vi "Unconstrained Logarithm Fit.vi"(0 "Y":dbl[](array[numeric]), 1 "base":dbl(ring)=2.71828 items=["e"=2.71828, "2"=2.0, "10"=10.0], 5 "X":dbl[](array[numeric]), 7 "Weight":dbl[](array[numeric]), 9 "tolerance":dbl=0.0001, 11 "method":T1 items=["Least Square", "Least Absolute Residual", "Bisquare"]) -> (4 "Best Logarithm Fit":dbl[](array[numeric]), 6 "amplitude":dbl, 8 "scale":dbl, 14 "residue":dbl, 15 "error":i32)   [LabVIEW 2017, in "NI_AALPro.lvlib"]
doc: "Returns the logarithmic fit of a data set (<B>X</B>, <B>Y</B>) using the Least Square, Least Absolute Residual, or Bisquare method."
uses:
  <vilib>/Analysis/NI_AALPro.lvlib
  <vilib>/Analysis/6fits.llb/Curve Fitting Criteria.ctl
panel:
  # "Logarithm Fit"
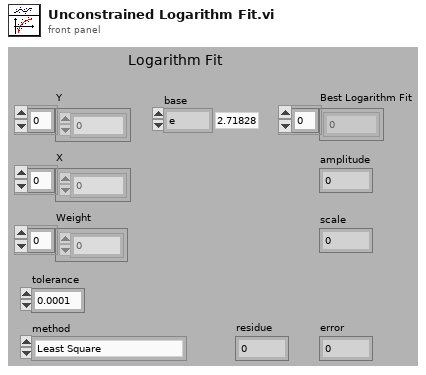
[diagram p1: front panel]
types:
  T1 = typedef "NI_AALPro.lvlib/Curve Fitting Criteria.ctl" = u16
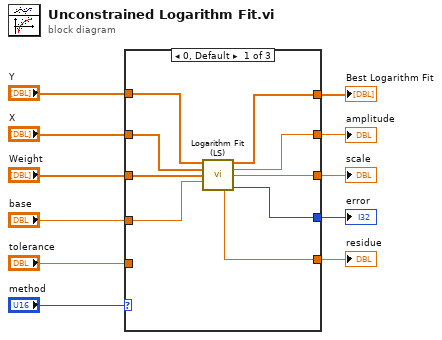
[diagram p0: block diagram]
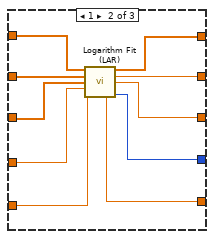
[diagram p2: hidden frame]
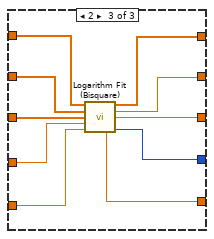
[diagram p3: hidden frame]
diagram:
  n1 = case shown="0, Default" "method" {
    tunnel: "Y" -> [w20 w30 w40]
    tunnel: "X" -> [w19 w29 w39]
    tunnel: "Weight" -> [w18 w28 w38]
    tunnel: "base" -> [w17 w27 w37]
    tunnel: [w16 w25 w35] -> w6
    tunnel: [w15 w24 w34] -> w5
    tunnel: [w14 w23 w33] -> w4
    tunnel: [w13 w22 w32] -> w3
    tunnel: [w12 w21 w31] -> w2
    tunnel: "tolerance" -> [_ w26 w36]
    frame 0, Default {
      n2 = call <vilib>:"Logarithm Fit (LS).vi"("Y"=w20, "X"=w19, "Weight"=w18, "base of logarithm"=w17) -> ("Best Logarithm Fit"=w16:dbl[], "amplitude"=w15:dbl, "scale"=w14:dbl, "residue"=w12:dbl, "error"=w13:i32)  [unwired: 7 out]
    }
    frame 1 {
      n3 = call <vilib>:"Logarithm Fit (LAR).vi"("Y"=w30, "X"=w29, "Weight"=w28, "base of logarithm"=w27, "tol"=w26) -> ("Best Logarithm Fit"=w25:dbl[], "amplitude"=w24:dbl, "scale"=w23:dbl, "residue"=w21:dbl, "error"=w22:i32)  [unwired: 6 out]
    }
    frame 2 {
      n4 = call <vilib>:"Logarithm Fit (Bisquare).vi"("Y"=w40, "X"=w39, "Weight"=w38, "base of logarithm"=w37, "tol"=w36) -> ("Best Logarithm Fit"=w35:dbl[], "amplitude"=w34:dbl, "scale"=w33:dbl, "residue"=w31:dbl, "error"=w32:i32)  [unwired: 6 out]
    }
  }
  "Best Logarithm Fit" <- w6
  "amplitude" <- w5
  "scale" <- w4
  "error" <- w3
  "residue" <- w2
